vi "configure.vi"(8 "error in (no error)":errorcluster, 11 "GenericPlugin in":refnum<class "TrajectoryAK101022Resonance.lvclass">) -> (0 "error out":errorcluster, 3 "GenericPlugin out":refnum<class "TrajectoryAK101022Resonance.lvclass">)   [LabVIEW 2010, in "TrajectoryAK101022Resonance.lvclass"]
doc: "The dynamic dispatch version of this VI loads and displays the configuration file associated with the plug-in object. The user modify and save the configuration data."
uses:
  TrajectoryAK101022Resonance.lvclass
  common/xcontrols/XComponentSpecification/XComponentSpecification/XComponentSpecification.xctl
  FPGAWrapper/GenericFPGAWrapper/GenericFPGAWrapper/GenericFPGAWrapper.lvclass
  TrajectoryAK101022Resonance.lvclass/TrajectoryAK101022Resonance.ctl
  common/classes/GenericComponent/GenericComponent/GenericComponent.lvclass
panel:
  in  "ETL current offset":dbl[unit]=0.06
  in  "ETL current to Hifo-Box conversion":dbl[unit]=20480.0
  in  "FPGAWrapper spec":T1(xcontrol)
  in  "objective magnification":dbl
  in  "FOVx":dbl[unit]
  in  "FOVy":dbl[unit]
  in  "resonance frequency":dbl[unit]
  in  "maximum y scanner value":dbl
  in  "maximum x scanner value":dbl
  in  "scan segment default":dbl
  in  "fly-back offset default":dbl
  in  "fly-forward offset default":dbl
  in  "no. of y-brake lines after flyback":i32
  in  "no. of y-flyback lines":i32
  in  "no. of y-brake lines before flyback":i32
  in  "cancelButton":bool
  in  "saveButton":bool
  out "configuration name":string
  # "Configure TrajectoryAK101022Resonance"
  # "FPGA wrapper"
  # "Note\nMeasure the Field Of View at zoom 1x and use the stage to measure left-to-right and top-to bottom.\nIndicate at which objective magnification this is measured."
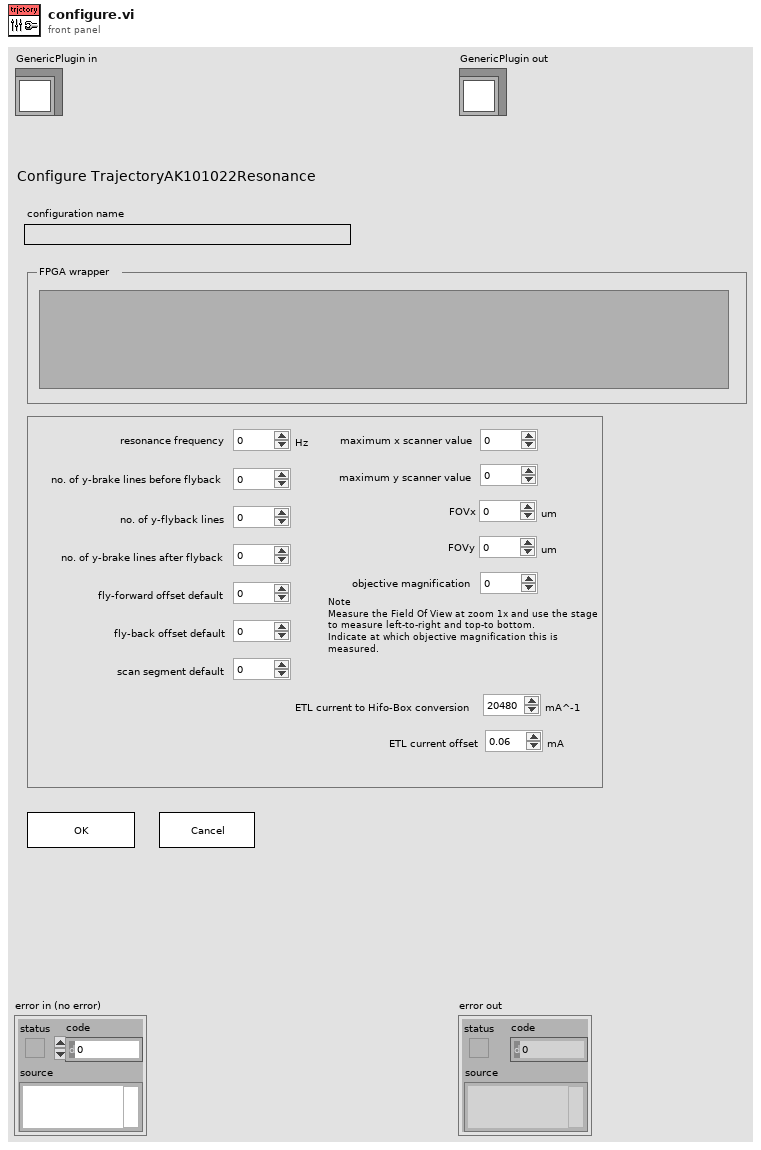
[diagram p1: front panel]
types:
  T1 = cluster{"class path":string, "configuration":string, "label":string, "settings name":string}
  T2 = typedef "plugin_specification.ctl" = cluster{"class path":string, "configuration":string, "label":string, "settings name":string}
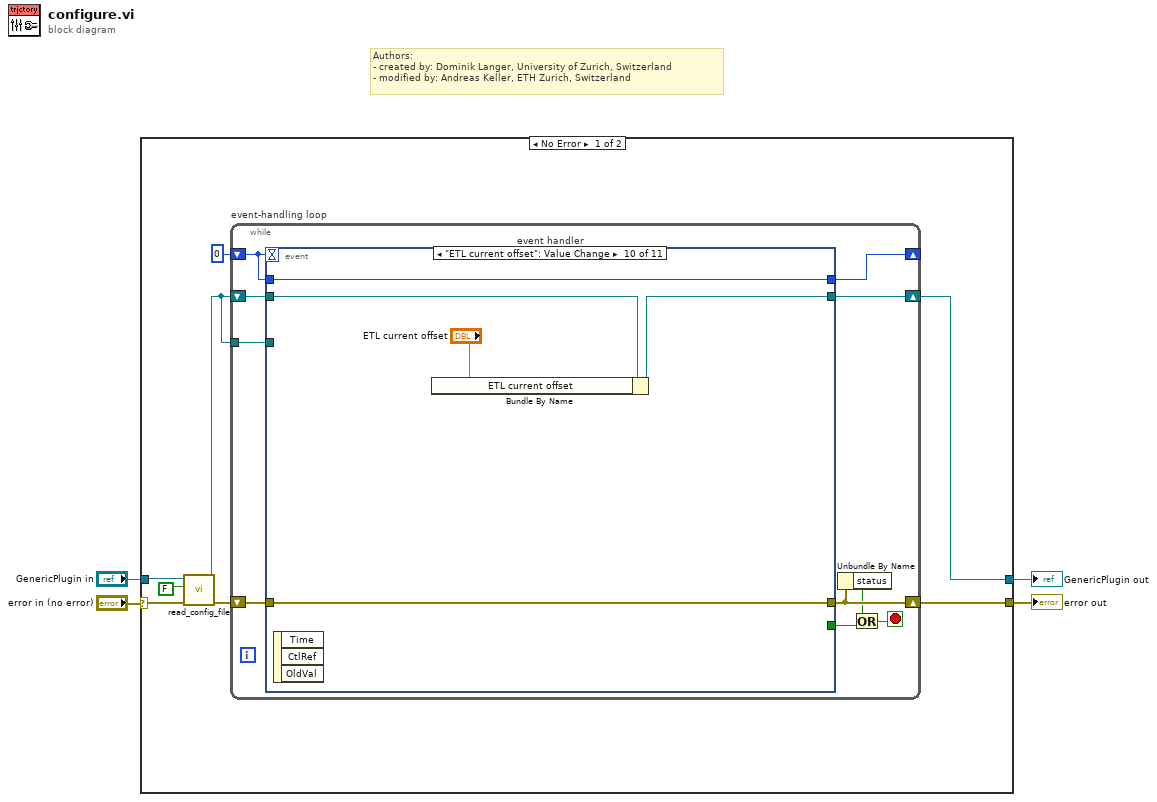
[diagram p0: block diagram]
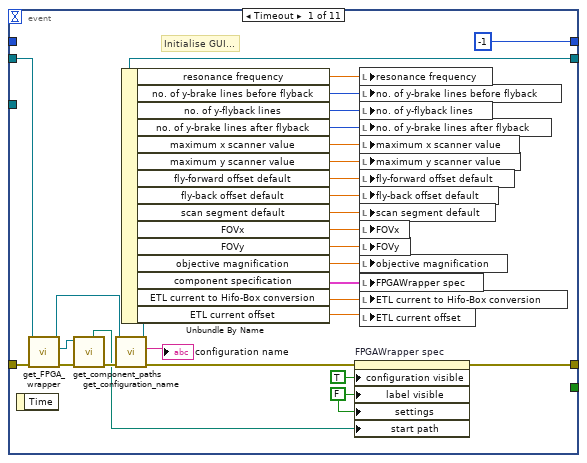
[diagram p2: hidden frame]
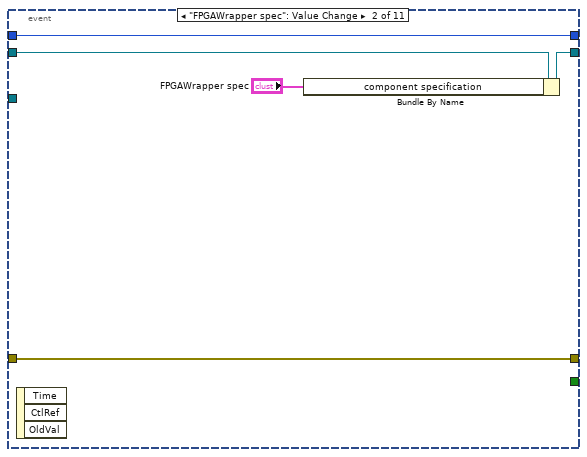
[diagram p3: hidden frame]
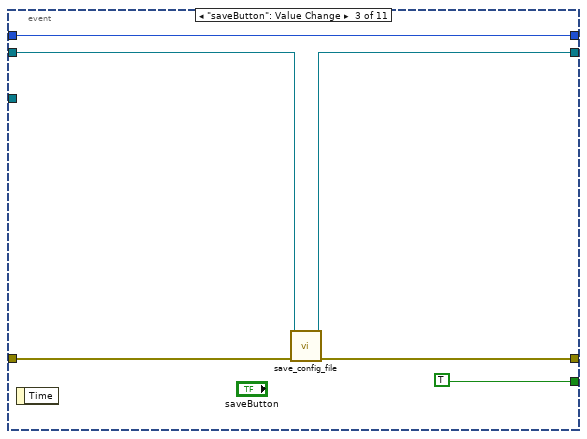
[diagram p4: hidden frame]
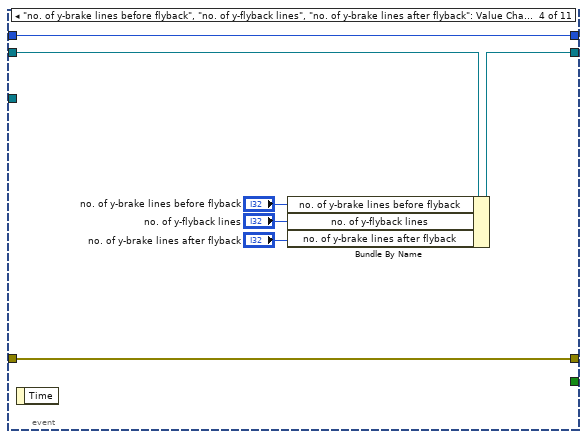
[diagram p5: hidden frame]
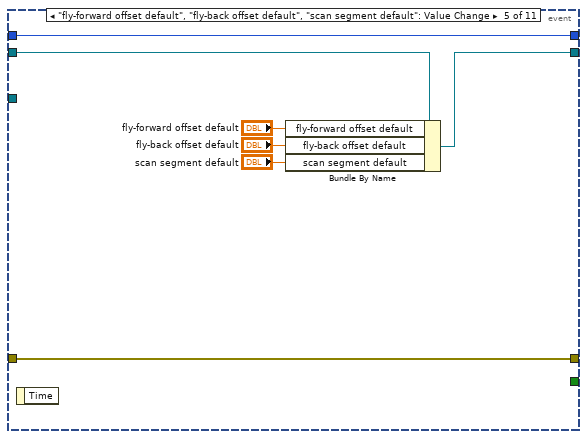
[diagram p6: hidden frame]
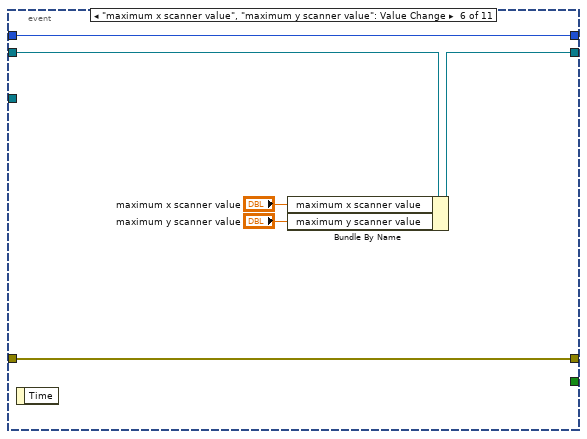
[diagram p7: hidden frame]
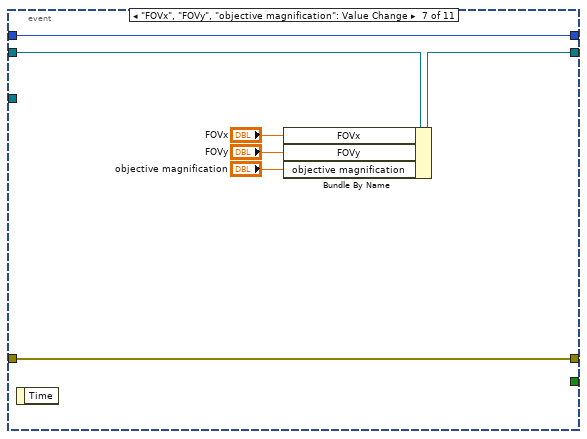
[diagram p8: hidden frame]
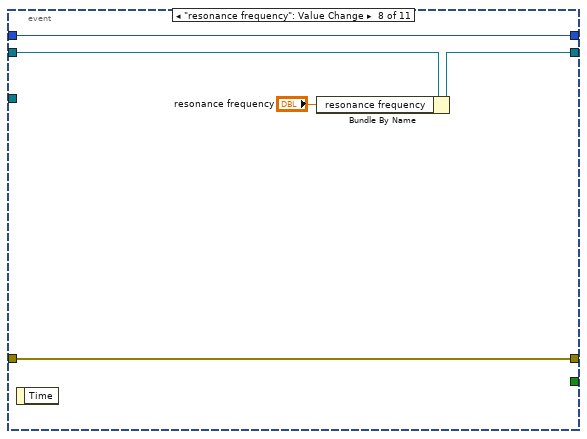
[diagram p9: hidden frame]
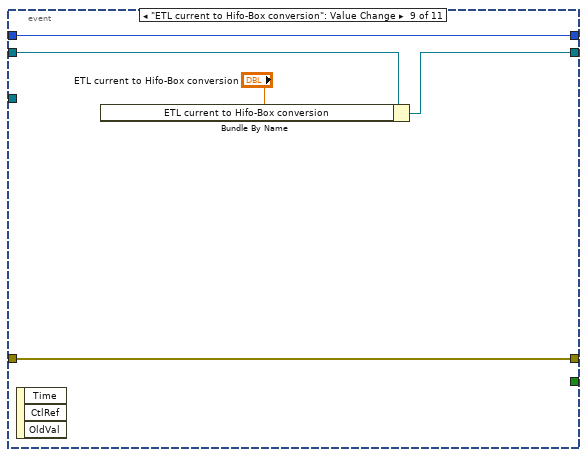
[diagram p10: hidden frame]
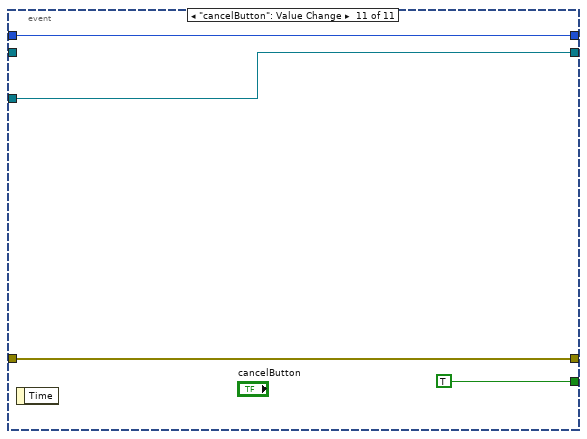
[diagram p11: hidden frame]
diagram:
  # "Authors: \n- created by: Dominik Langer, University of Zurich, Switzerland\n- modified by: Andreas Keller, ETH Zurich, Switzerland"
  n1 = case shown="No Error" "error in (no error)" {
    selector: "error in (no error)" -> [w7 w109]
    tunnel: [w6 w109] -> w3
    tunnel: [w5 w110] -> w1
    tunnel: "GenericPlugin in" -> [w8 w110]
    frame No Error {
      n2 = call-dynamic "read_config_file.vi"("error in (no error)"=w7, "force load?"=FALSE, "GenericPlugin in"=w8) -> ("error out"=w12:errorcluster, "GenericPlugin out"=w11:refnum<class "TrajectoryAK101022Resonance.lvclass">)  [unwired: 7 in]
      n3 = while "event-handling loop" {
        shift-right: [w19] -> w6
        shift-left: w12 -> [w22]
        shift-right: [w20] -> w5
        shift-left: w11 -> [w21]
        tunnel: w11 -> [w15]
        shift-right: [w13] -> _
        shift-left: 0 -> [w14]
        stop <- w16 stop-if-true
        n4 = event "event handler" shown="[9] \"ETL current offset\": Value Change" {
          selector: _ -> [_ _ _ _ _ _ _ _ _ _ _]
          dyn-events: _ -> [_ _ _ _ _ _ _ _ _ _ _]
          timeout: w14 -> [_ _ _ _ _ _ _ _ _ _ _]
          tunnel: w22 -> [w33 w56 w61 w69 w76 w82 w89 w94 w99 w104 w108]
          tunnel: [w28 w56 w60 w69 w76 w82 w89 w94 w99 w104 w108] -> w19
          tunnel: w21 -> [w32 w53 w59 w68 w74 w81 w87 w93 w97 w102 _]
          tunnel: [w50 w52 w58 w67 w73 w80 w86 w92 w96 w101 w106] -> w20
          tunnel: [_ _ TRUE _ _ _ _ _ _ _ TRUE] -> w18
          tunnel: w15 -> [_ _ _ _ _ _ _ _ _ _ w106]
          tunnel: [-1 w55 w57 w66 w75 w79 w88 w91 w98 w103 w105] -> w13
          tunnel: w14 -> [_ w55 w57 w66 w75 w79 w88 w91 w98 w103 w105]
          event Timeout {
            w35 = FALSE ("label visible")
            # "Initialise GUI..."
            n5 = event-data() -> ()  [unwired: 1 in, 1 out]
            n6 = call-dynamic "get_FPGA_wrapper.vi"("error in (no error)"=w33, "TrajectoryMG100122GenericFPGA in"=w32) -> ("error out"=w31:errorcluster, "GenericFPGAWrapper.lvclass"=w26:refnum<class "GenericFPGAWrapper.lvclass">, "TrajectoryMG100122GenericFPGA out"=w25:refnum<class "TrajectoryAK101022Resonance.lvclass">)  [unwired: 7 in]
            n7 = call-dynamic "get_component_paths.vi"("error in (no error)"=w31, "GenericComponent in"=w26) -> ("error out"=w30:errorcluster, "component type directory"=w27:path)  [unwired: 4 in, 4 out]
            n8 = call "get_configuration_name.vi"("error in (no error)"=w30, "GenericPlugin.lvclass in"=w25) -> ("error out"=w29:errorcluster, "configuration name"=→"configuration name":string, "GenericPlugin.lvclass out"=w50:refnum<class "TrajectoryAK101022Resonance.lvclass">)  [unwired: 7 in]
            n9 = Unbundle By Name(w50) -> ("resonance frequency"=w48:dbl[unit], "no. of y-brake lines before flyback"=w47:i32, "no. of y-flyback lines"=w46:i32, "no. of y-brake lines after flyback"=w45:i32, "maximum x scanner value"=w44:dbl, "maximum y scanner value"=w43:dbl, "fly-forward offset default"=w42:dbl, "fly-back offset default"=w41:dbl, "scan segment default"=w40:dbl, "FOVx"=w39:dbl[unit], "FOVy"=w38:dbl[unit], "objective magnification"=w37:dbl, "component specification"=w34:T2, "ETL current to Hifo-Box conversion"=w24:dbl[unit], "ETL current offset"=w23:dbl[unit])
            n10 = property on="FPGAWrapper spec" class="XComponentSpecification (strict"(error in=w29, "configuration visible"=TRUE, "label visible"=w35, "settings"=w35, "start path"=w27) -> (error out=w28:errorcluster)  [unwired: 1 in, 1 out]
            n11 = local write "resonance frequency"(w48) -> ()
            n12 = local write "no. of y-brake lines before flyback"(w47) -> ()
            n13 = local write "no. of y-flyback lines"(w46) -> ()
            n14 = local write "no. of y-brake lines after flyback"(w45) -> ()
            n15 = local write "maximum x scanner value"(w44) -> ()
            n16 = local write "maximum y scanner value"(w43) -> ()
            n17 = local write "fly-forward offset default"(w42) -> ()
            n18 = local write "fly-back offset default"(w41) -> ()
            n19 = local write "scan segment default"(w40) -> ()
            n20 = local write "FOVx"(w39) -> ()
            n21 = local write "FOVy"(w38) -> ()
            n22 = local write "objective magnification"(w37) -> ()
            n23 = local write "FPGAWrapper spec"(w34) -> ()
            n24 = local write "ETL current to Hifo-Box conversion"(w24) -> ()
            n25 = local write "ETL current offset"(w23) -> ()
          }
          event "FPGAWrapper spec": Value Change {
            n26 = event-data() -> ()  [unwired: 1 in, 3 out]
            n27 = Bundle By Name(cluster=w53, "component specification"="FPGAWrapper spec") -> (w52:refnum<class "TrajectoryAK101022Resonance.lvclass">)
          }
          event "saveButton": Value Change {
            n28 = event-data() -> ()  [unwired: 1 in, 1 out]
            n29 = call-dynamic "save_config_file.vi"("error in (no error)"=w61, "GenericPlugin in"=w59) -> ("error out"=w60:errorcluster, "GenericPlugin out"=w58:refnum<class "TrajectoryAK101022Resonance.lvclass">)  [unwired: 8 in]
          }
          event "no. of y-brake lines before flyback", "no. of y-flyback lines", "no. of y-brake lines after flyback": Value Change {
            n30 = event-data() -> ()  [unwired: 1 in, 1 out]
            n31 = Bundle By Name(cluster=w68, "no. of y-brake lines before flyback"="no. of y-brake lines before flyback", "no. of y-flyback lines"="no. of y-flyback lines", "no. of y-brake lines after flyback"="no. of y-brake lines after flyback") -> (w67:refnum<class "TrajectoryAK101022Resonance.lvclass">)
          }
          event "fly-forward offset default", "fly-back offset default", "scan segment default": Value Change {
            n32 = event-data() -> ()  [unwired: 1 in, 1 out]
            n33 = Bundle By Name(cluster=w74, "fly-forward offset default"="fly-forward offset default", "fly-back offset default"="fly-back offset default", "scan segment default"="scan segment default") -> (w73:refnum<class "TrajectoryAK101022Resonance.lvclass">)
          }
          event "maximum x scanner value", "maximum y scanner value": Value Change {
            n34 = event-data() -> ()  [unwired: 1 in, 1 out]
            n35 = Bundle By Name(cluster=w81, "maximum x scanner value"="maximum x scanner value", "maximum y scanner value"="maximum y scanner value") -> (w80:refnum<class "TrajectoryAK101022Resonance.lvclass">)
          }
          event "FOVx", "FOVy", "objective magnification": Value Change {
            n36 = event-data() -> ()  [unwired: 1 in, 1 out]
            n37 = Bundle By Name(cluster=w87, "FOVx"="FOVx", "FOVy"="FOVy", "objective magnification"="objective magnification") -> (w86:refnum<class "TrajectoryAK101022Resonance.lvclass">)
          }
          event "resonance frequency": Value Change {
            n38 = event-data() -> ()  [unwired: 1 in, 1 out]
            n39 = Bundle By Name(cluster=w93, "resonance frequency"="resonance frequency") -> (w92:refnum<class "TrajectoryAK101022Resonance.lvclass">)
          }
          event "ETL current to Hifo-Box conversion": Value Change {
            n40 = event-data() -> ()  [unwired: 1 in, 3 out]
            n41 = Bundle By Name(cluster=w97, "ETL current to Hifo-Box conversion"="ETL current to Hifo-Box conversion") -> (w96:refnum<class "TrajectoryAK101022Resonance.lvclass">)
          }
          event "ETL current offset": Value Change {
            n42 = event-data() -> ()  [unwired: 1 in, 3 out]
            n43 = Bundle By Name(cluster=w102, "ETL current offset"="ETL current offset") -> (w101:refnum<class "TrajectoryAK101022Resonance.lvclass">)
          }
          event "cancelButton": Value Change {
            n44 = event-data() -> ()  [unwired: 1 in, 1 out]
          }
        }
        n45 = Unbundle By Name(w19) -> ("status"=w17:bool)
        n46 = Or(x=w17, y=w18) -> (x .or. y?=w16:bool)
      }
    }
    frame Error {
    }
  }
  "error out" <- w3
  "GenericPlugin out" <- w1
